vi "log_data.vi"(0 "Log File":path, 1 "Carrier amplitudes":cdb[][][](array[numeric]) format="%#_4g", 3 "Ref carrier ampl":cdb[][][](array[numeric])=[[[1.0+0.0i, 1.0+0.0i, 1.0+0.0i], [1.0+0.0i, 1.0+0.0i, 1.0+0.0i]], [[1.0+0.0i, 1.0+0.0i, 1.0+0.0i], [1.0+0.0i, 1.0+0.0i, 1.0+0.0i]]] format="%#_3p", 5 "Start Logging":bool, 9 "Stop Logging":bool, 11 "Time Stamp":timestamp, 12 "Trace info in":T3, 13 "Log mode":T1, 14 "Modulation info":T2={"Fs full"=0.0, "Fs high"=0.0, "Fs low"=0.0, "Read size"=5000, "FFT size low"=5000, "df low"=5000.0, "High carriers"=[], "Low carriers"=[], "Hi channels at low"=[7]} {"Hi channels at low" min=0 step=1; "Low carriers" format="%#_6p"; "High carriers" format="%#_6p"}) -> (4 "Logging":bool)   [LabVIEW 2014]
doc: "Converts an array of data to a row of tab-separated columns, prepends the timestamp column, and terminates each row with the end of line character."
uses:
  trace_info.ctl
  trace_channel.ctl
  ilemt_status.ctl
  modulation_info.ctl
  log_mode.ctl
  ilemt_globals.vi
panel:
  out "Result string":string
  # "Debug display:"
  # "Note that each dumped row is a couping matrix in column major format, where rows are source axes and columns are sensor axes. See comment in coupling_to_string for more details."
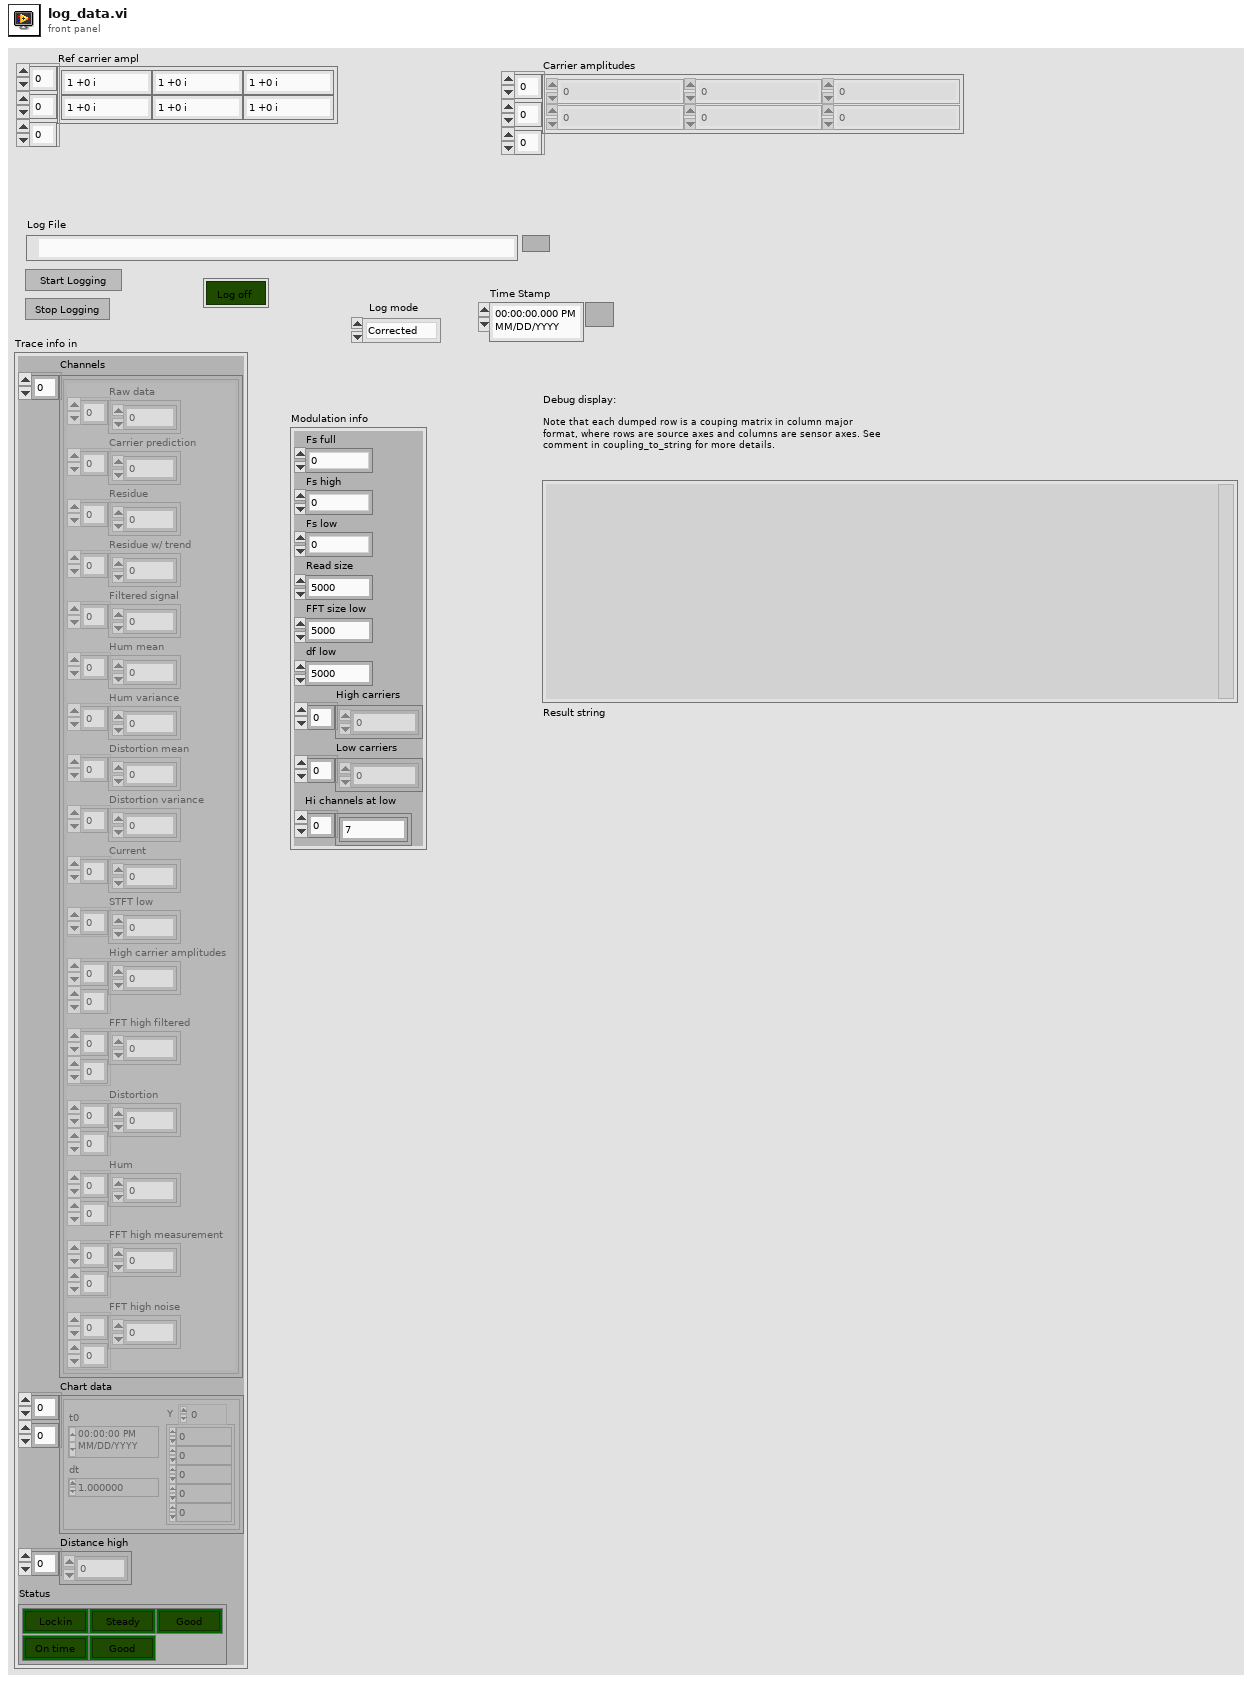
[diagram p1: front panel]
types:
  T1 = typedef "log_mode.ctl" = enum16{"Corrected", "Raw"}
  T2 = typedef "modulation_info.ctl" = cluster{"Fs full":dbl, "Fs high":dbl, "Fs low":dbl, "Read size":i32, "FFT size low":i32, "df low":dbl, "High carriers":dbl[], "Low carriers":dbl[], "Hi channels at low":i32[]}
  T3 = typedef "trace_info.ctl" = cluster{"Channels":T4[], "Chart data":waveform(dbl)[][], "Distance high":dbl[], "Status":T5}
  T4 = typedef "trace_channel.ctl" = cluster{"Raw data":dbl[], "Carrier prediction":dbl[], "Residue":dbl[], "Residue w/ trend":dbl[], "Filtered signal":dbl[], "Hum mean":dbl[], "Hum variance":dbl[], "Distortion mean":dbl[], "Distortion variance":dbl[], "Current":dbl[], "STFT low":cdb[], "High carrier amplitudes":cdb[][], "FFT high filtered":cdb[][], "Distortion":cdb[][], "Hum":cdb[][], "FFT high measurement":cdb[][], "FFT high noise":dbl[][]}
  T5 = typedef "ilemt_status.ctl" = cluster{"Unlocked":bool, "Impulse":bool, "NaN":bool, "Backlog":bool, "Clipping":bool}
  T6 = enum16{"open", "replace", "create", "open or create", "replace or create", "replace or create with confirmation"}
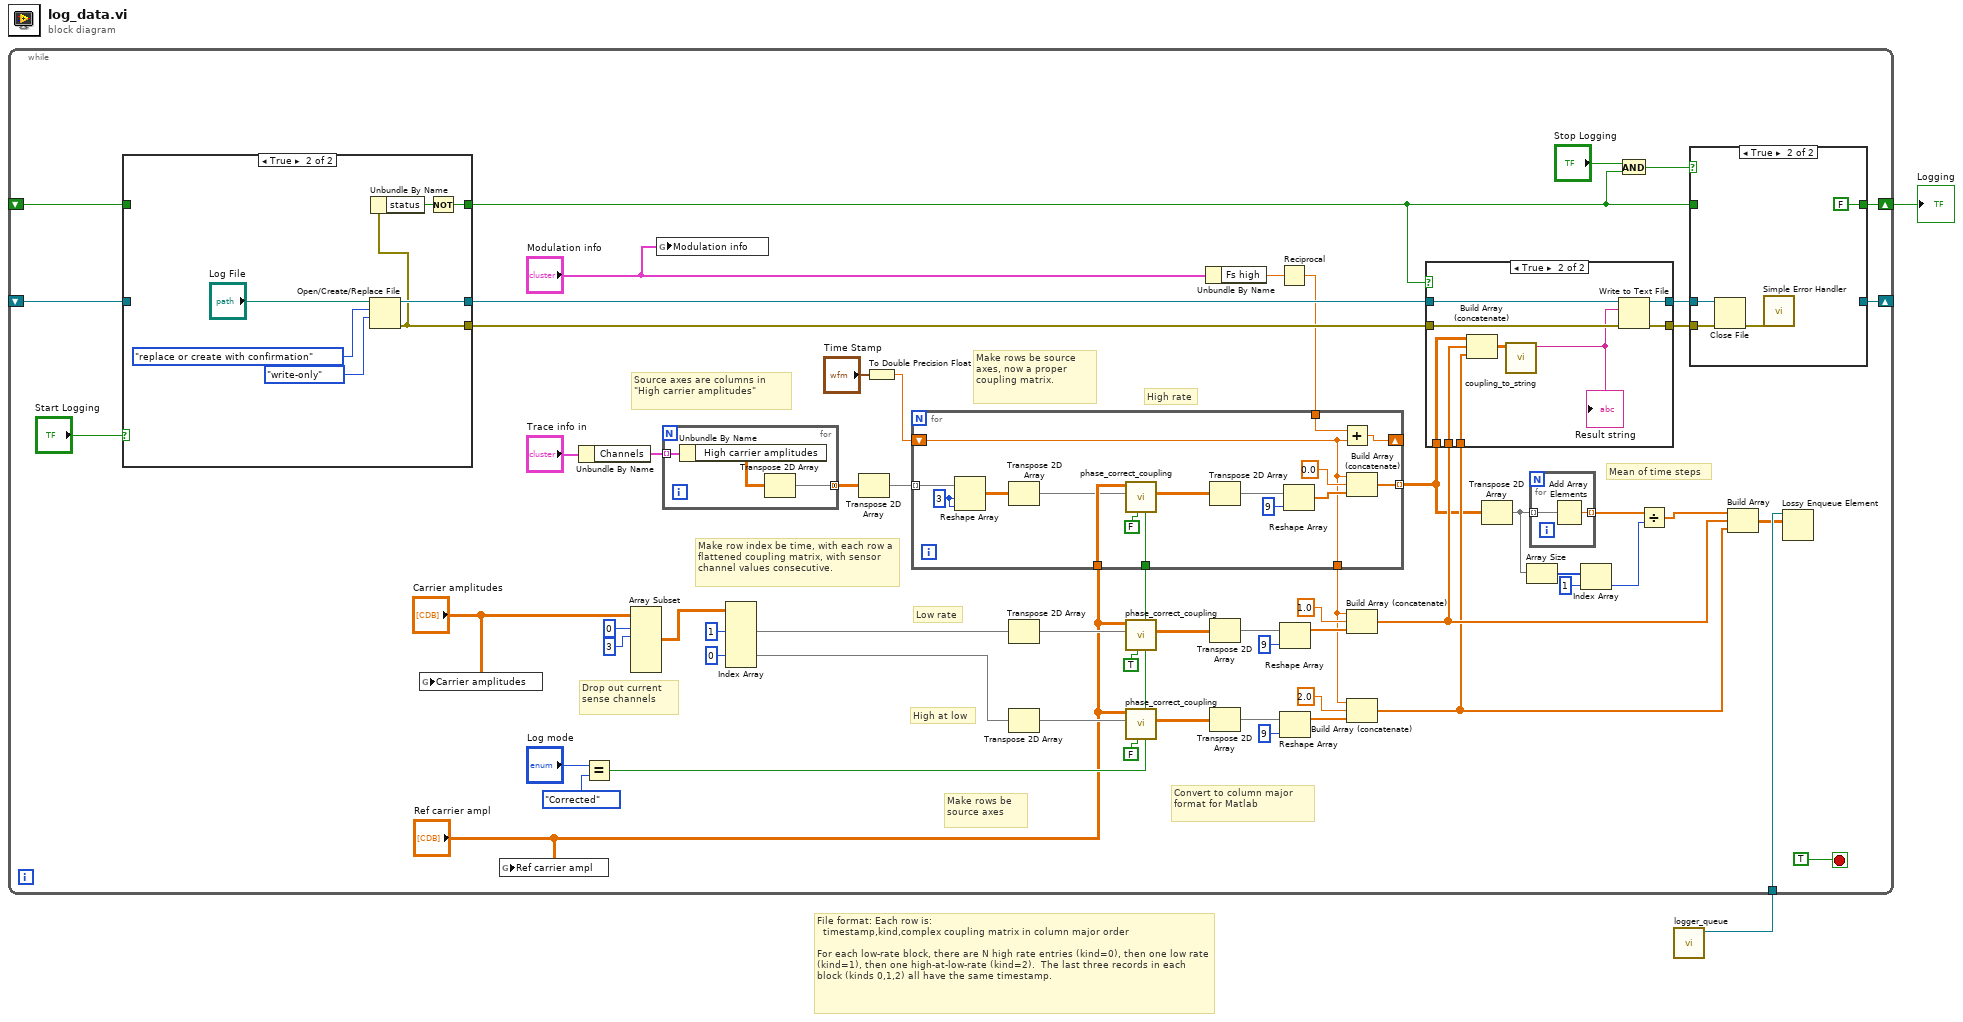
[diagram p0: block diagram]
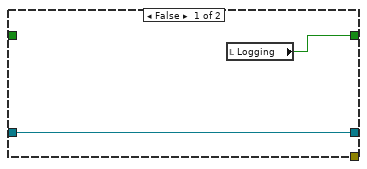
[diagram p4: hidden frame]
diagram:
  # "File format: Each row is:\n  timestamp,kind,complex coupling matrix in column major order\n\nFor each low-rate block, there are N high rate entries (kind=0), then one low rate (kind=1), then one high-at-low-rate (kind=2).  The last three records in each block (kinds 0,1,2) all have the same timestamp."
  n1 = call "logger_queue.vi"() -> ("queue out"=w1:refnum<queue>)  [unwired: 10 in, 1 out]
  n2 = while {
    shift-right: [w58] -> _
    shift-left: _ -> [w59]
    shift-right: [w51] -> w2
    shift-left: _ -> [w52]
    tunnel: w1 -> [w14]
    stop <- TRUE stop-if-true
    # "Mean of time steps"
    # "Make rows be source axes, now a proper coupling matrix."
    # "Make row index be time, with each row a flattened coupling matrix, with sensor channel values consecutive."
    # "Source axes are columns in \"High carrier amplitudes\""
    # "Make rows be source axes"
    # "Convert to column major format for Matlab"
    # "High at low"
    # "Drop out current sense channels"
    # "High rate"
    # "Low rate"
    n3 = case shown="True" "Start Logging" {
      tunnel: [w102 w109] -> w61
      tunnel: [_ w105] -> w62
      tunnel: w59 -> [w102 _]
      tunnel: [w101 w103] -> w17
      tunnel: w52 -> [_ _]
      frame False {
        n4 = local read "Logging"() -> (w101:bool)
      }
      frame True {
        n5 = Open/Create/Replace File(file path (use dialog)="Log File", operation (0:open)=T6."replace or create with confirmation", access (0:read/write)=enum16{"read/write", "read-only", "write-only"}."write-only") -> (refnum out=w109:refnum<file>, error out=w105:errorcluster)  [unwired: 2 in, 2 out]
        n6 = Unbundle By Name(w105) -> ("status"=w104:bool)
        n7 = Not(x=w104) -> (.not. x?=w103:bool)
      }
    }
    n8 = global write "ilemt_globals.vi" "Carrier amplitudes"("Carrier amplitudes") -> ()
    n9 = global write "ilemt_globals.vi" "Ref carrier ampl"("Ref carrier ampl") -> ()
    n10 = Unbundle By Name("Trace info in") -> ("Channels"=w49:T4[])
    n11 = Equal?(x="Log mode", y=log_mode."Corrected") -> (x = y?=w20:bool)
    n12 = Array Subset(array="Carrier amplitudes", index (dim 0)=0 ("index"), length (dim 0)=3 ("length")) -> (w30:cdb[][][])  [unwired: 4 in]
    n13 = global write "ilemt_globals.vi" "Modulation info"("Modulation info") -> ()
    n14 = for {
      tunnel: w49 -> [w94] mode=indexing
      tunnel: [w93] -> w50 mode=concatenating
      n15 = Unbundle By Name(w94) -> ("High carrier amplitudes"=w92:cdb[][])
      n16 = Transpose 2D Array(2D array=w92) -> (transposed array=w93:cdb[][])
    }
    n17 = Index Array(array=w30, index (dim 1) #1=1 ("disabled index (row)"), index (dim 1) #2=0 ("disabled index (row)")) -> (element #1=w28:cdb[][], element #2=w19:cdb[][])  [unwired: 4 in]
    n18 = Transpose 2D Array(2D array=w50) -> (transposed array=w47:cdb[][])
    n19 = To Double Precision Float(number="Time Stamp") -> (double precision float=w34:dbl)
    n20 = Transpose 2D Array(2D array=w28) -> (transposed array=w42:cdb[][])
    n21 = Transpose 2D Array(2D array=w19) -> (transposed array=w22:cdb[][])
    n22 = call "phase_correct_coupling.vi"("Really correct?"=w20, "Is low?"=TRUE, "Complex coupling"=w42, "Ref carrier ampl"="Ref carrier ampl") -> ("Phase corrected coupling"=w38:cdb[][])  [unwired: 6 in, 1 out]
    n23 = call "phase_correct_coupling.vi"("Really correct?"=w20, "Is low?"=FALSE, "Complex coupling"=w22, "Ref carrier ampl"="Ref carrier ampl") -> ("Phase corrected coupling"=w26:cdb[][])  [unwired: 6 in, 1 out]
    n24 = Unbundle By Name("Modulation info") -> ("Fs high"=w36:dbl)
    n25 = Transpose 2D Array(2D array=w38) -> (transposed array=w37:cdb[][])
    n26 = Transpose 2D Array(2D array=w26) -> (transposed array=w27:cdb[][])
    n27 = Reciprocal(x=w36) -> (1/x=w33:dbl)
    n28 = for {
      tunnel: w47 -> [w90] mode=indexing
      tunnel: [w85] -> w7 mode=indexing
      tunnel: "Ref carrier ampl" -> [w77]
      shift-right: [w83] -> _
      shift-left: w34 -> [w81]
      tunnel: w33 -> [w84]
      tunnel: [w81] -> w18
      tunnel: w20 -> [w82]
      w89 = 3 ("dimension size")
      n29 = Reshape Array(w90, w89, w89) -> (w78:cdb[][])
      n30 = Transpose 2D Array(2D array=w78) -> (transposed array=w76:cdb[][])
      n31 = call "phase_correct_coupling.vi"("Really correct?"=w82, "Is low?"=FALSE, "Complex coupling"=w76, "Ref carrier ampl"=w77) -> ("Phase corrected coupling"=w80:cdb[][])  [unwired: 6 in, 1 out]
      n32 = Transpose 2D Array(2D array=w80) -> (transposed array=w79:cdb[][])
      n33 = Reshape Array(w79, 9 ("dimension size")) -> (w87:cdb[])
      n34 = Add(x=w84, y=w81) -> (x+y=w83:dbl)
      n35 = Build Array (concatenate)(w81, 0.0, w87) -> (w85:cdb[])
    }
    n36 = Reshape Array(w37, 9 ("dimension size")) -> (w41:cdb[])
    n37 = Reshape Array(w27, 9 ("dimension size")) -> (w23:cdb[])
    n38 = Build Array (concatenate)(w18, 1.0, w41) -> (w16:cdb[])
    n39 = Build Array (concatenate)(w18, 2.0, w23) -> (w15:cdb[])
    n40 = case shown="True" w17 {
      tunnel: w62 -> [w65 w75]
      tunnel: w61 -> [w66 w74]
      tunnel: [w66 w73] -> w57
      tunnel: [w65 w72] -> w56
      tunnel: w16 -> [_ w71]
      tunnel: w7 -> [_ w70]
      tunnel: w15 -> [_ w67]
      frame False {
      }
      frame True {
        n41 = Build Array (concatenate)(w70, w71, w67) -> (w69:cdb[][])
        n42 = call "coupling_to_string.vi"("Coupling data"=w69) -> ("Result string"=w68:string)  [unwired: 10 in]
        "Result string" <- w68
        n43 = Write to Text File(file (use dialog)=w74, text=w68, error in=w75) -> (refnum out=w73:refnum<file>, error out=w72:errorcluster)  [unwired: 1 in, 1 out]
      }
    }
    n44 = Transpose 2D Array(2D array=w7) -> (transposed array=w3:cdb[][])
    n45 = Array Size(array=w3) -> (size(s)=w6:i32[])
    n46 = for {
      tunnel: w3 -> [w64] mode=indexing
      tunnel: [w63] -> w8 mode=indexing
      n47 = Add Array Elements(numeric array=w64) -> (sum=w63:cdb)
    }
    n48 = Index Array(array=w6, index=1) -> (element=w4:i32)
    n49 = And(x="Stop Logging", y=w17) -> (x .and. y?=w55:bool)
    n50 = Divide(x=w8, y=w4) -> (x/y=w9:cdb[])
    n51 = case shown="True" w55 {
      tunnel: [w96 _] -> w58
      tunnel: w57 -> [w96 w99]
      tunnel: w56 -> [_ w98]
      tunnel: [w95 FALSE] -> w51
      tunnel: w17 -> [w95 _]
      frame False {
      }
      frame True {
        n52 = Close File(refnum=w99, error in=w98) -> (error out=w100:errorcluster)  [unwired: 1 out]
        n53 = call <vilib>:"Simple Error Handler.vi"("error in (no error)"=w100) -> ()  [unwired: 1 in, 8 out]
      }
    }
    n54 = Build Array(w9, w16, w15) -> (w13:cdb[][])
    n55 = Lossy Enqueue Element(queue=w14, element=w13) -> ()  [unwired: 1 in, 4 out]
  }
  "Logging" <- w2
